vi "ShapeDectect.vi"(8 "error in (no error)":errorcluster, 9 "ROI Descriptor":T2, 10 "SetParameter":T4={"Enum_ShapeType"=enum."Circles", "MaxParticle"=1, "Descriptor"={"Set 1"=100.0, "Set 2"=10.0, "Set 3"=200.0, "Set 4"=10.0}, "Match Options"={"Rotation"=TRUE, "Scale"=FALSE, "Occlusion"=FALSE, "Range Settings"=[{"Match Constraints"=0, "Min"=0.0, "Max"=360.0}]}, "Curve Parameters"={"Extraction Mode"=0, "Edge Threshold"=75, "Edge Filter Size"=1, "Min Length"=25, "Row Search Step Size"=15, "Col Search Step Size"=15, "Max Endpoint Gap"=10, "Closed"=FALSE, "Subpixel"=FALSE}, " score"=500.0} {"score" format="%#_15g"; "Curve Parameters"."Extraction Mode" items=["Normal", "Uniform Regions"]; "Curve Parameters"."Edge Filter Size" items=["Fine", "Normal"]; "Match Options"."Range Settings"."Match Constraints" items=["Rotation Angle (degrees)", "Scale Factor (%)", "Occlusion (%)"]}, 11 "Image In":T3) -> (0 "error out":errorcluster, 1 "DectectItem":i32, 2 "ResultOut":variant, 3 "Image Out":T3)   [LabVIEW 2019]
uses:
  <vilib>/vision/Image Controls.llb/IMAQ Image.ctl
  Controls/ShapeDectect/Analysis_ShapeDectect_Parameter.ctl
  Controls/ShapeDectect/V_ShapeDectectFinalResult.ctl
  <vilib>/vision/NI_Vision_Development_Module.lvlib
panel:
  in  "Shapedectect Result Out":T1
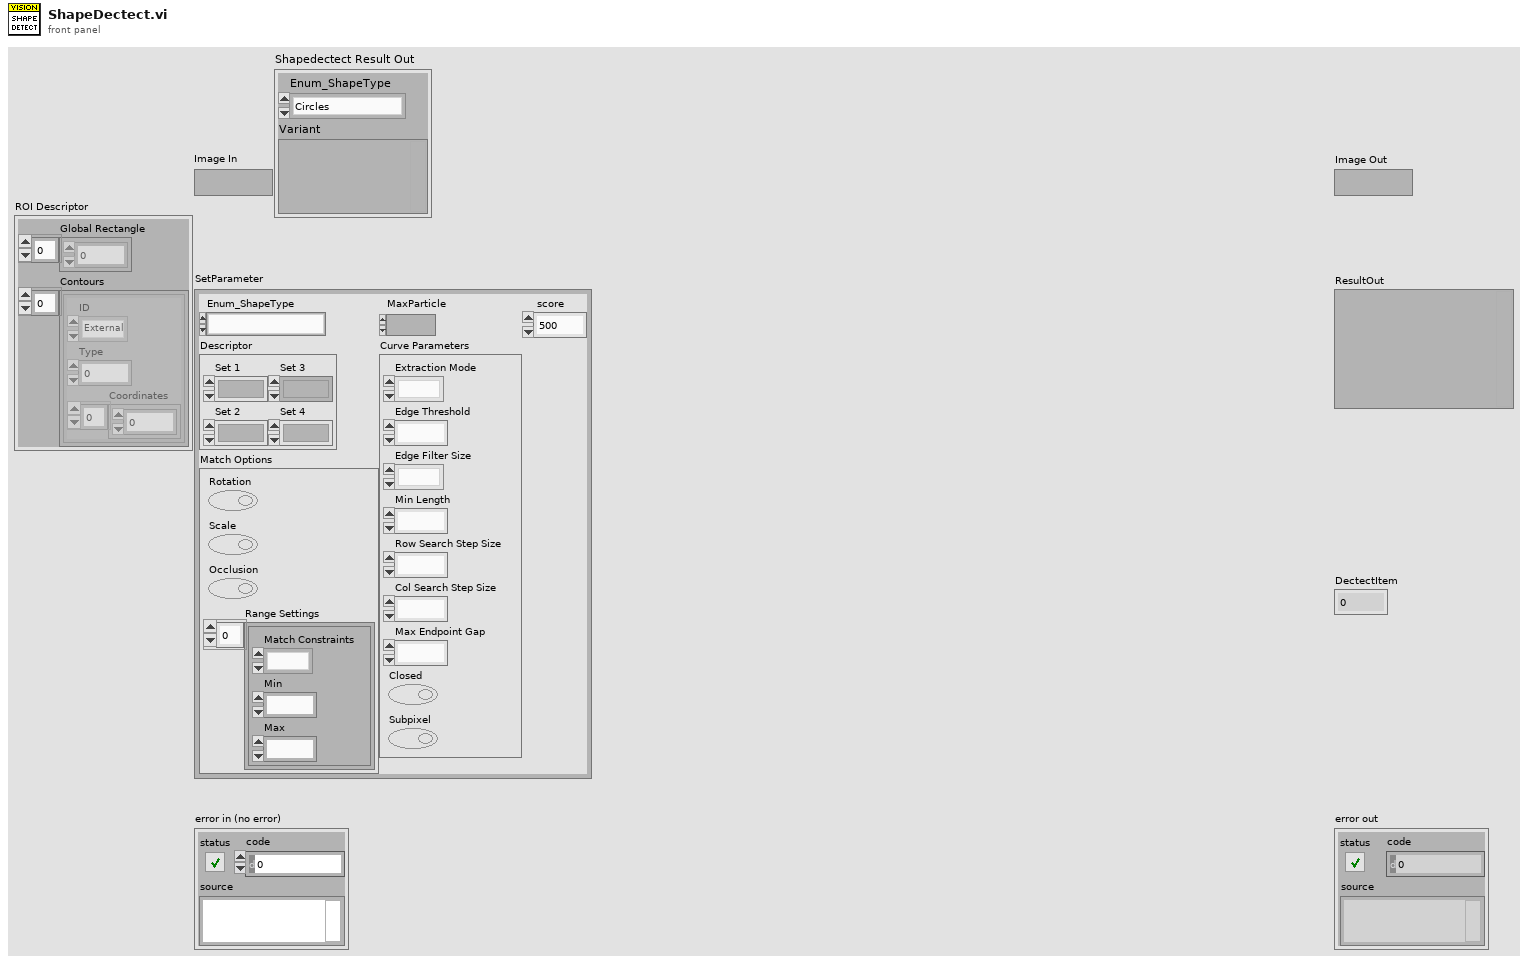
[diagram p1: front panel]
types:
  T1 = typedef "V_ShapeDectectFinalResult.ctl" = cluster{"Enum_ShapeType":enum16{"Circles", "Ellipses", "Lines", "Rectangles"}, "Variant":variant}
  T2 = cluster{"Global Rectangle":i32[], "Contours":cluster{"ID":enum32{"External", "Internal"}, "Type":u32, "Coordinates":i32[]}[]}
  T3 = typedef "IMAQ Image.ctl" = refnum<image>
  T4 = typedef "Analysis_ShapeDectect_Parameter.ctl" = cluster{"Enum_ShapeType":enum16{"Circles", "Ellipses", "Lines", "Rectangles"}, "MaxParticle":i32, "Descriptor":cluster{"Set 1":dbl, "Set 2":dbl, "Set 3":dbl, "Set 4":dbl}, "Match Options":cluster{"Rotation":bool, "Scale":bool, "Occlusion":bool, "Range Settings":cluster{"Match Constraints":u32, "Min":dbl, "Max":dbl}[]}, "Curve Parameters":cluster{"Extraction Mode":u32, "Edge Threshold":i32, "Edge Filter Size":u32, "Min Length":i32, "Row Search Step Size":i32, "Col Search Step Size":i32, "Max Endpoint Gap":i32, "Closed":bool, "Subpixel":bool}, " score":dbl}
  T5 = cluster{"Rectangles":cluster{"Corners":cluster{"X":sgl, "Y":sgl}[], "Angle":dbl, "Width":dbl, "Height":dbl, "Score":dbl}[], "Rectangles Calibrated":cluster{"Corners":cluster{"X":sgl, "Y":sgl}[], "Angle":dbl, "Width":dbl, "Height":dbl, "Score":dbl}[]}
  T6 = cluster{"Lines":cluster{"Start Point":cluster{"X":sgl, "Y":sgl}, "End Point":cluster{"X":sgl, "Y":sgl}, "Length":dbl, "Angle":dbl, "Score":dbl}[], "Lines Calibrated":cluster{"Start Point":cluster{"X":sgl, "Y":sgl}, "End Point":cluster{"X":sgl, "Y":sgl}, "Length":dbl, "Orientation":dbl, "Score":dbl}[]}
  T7 = cluster{"Pixel":cluster{"Position":cluster{"X":sgl, "Y":sgl}, "Angle":dbl, "Major Radius":dbl, "Minor Radius":dbl, "Score":dbl}[], "Ellipses (Calibrated)":cluster{"Position":cluster{"X":sgl, "Y":sgl}, "Orientation":dbl, "Major Radius":dbl, "Minor Radius":dbl, "Score":dbl}[]}
  T8 = cluster{"Circles":cluster{"Position":cluster{"X":sgl, "Y":sgl}, "Radius":dbl, "Score":dbl}[], "Circles (Calibrated)":cluster{"Position":cluster{"X":sgl, "Y":sgl}, "Radius":dbl, "Score":dbl}[]}
  T9 = enum16{"Circles", "Ellipses", "Lines", "Rectangles"}
  T10 = cluster{"Set 1":dbl, "Set 2":dbl, "Set 3":dbl, "Set 4":dbl}
  T11 = cluster{"Rotation":bool, "Scale":bool, "Occlusion":bool, "Range Settings":cluster{"Match Constraints":u32, "Min":dbl, "Max":dbl}[]}
  T12 = cluster{"Extraction Mode":u32, "Edge Threshold":i32, "Edge Filter Size":u32, "Min Length":i32, "Row Search Step Size":i32, "Col Search Step Size":i32, "Max Endpoint Gap":i32, "Closed":bool, "Subpixel":bool}
  T13 = cluster{"Position":cluster{"X":sgl, "Y":sgl}, "Radius":dbl, "Score":dbl}
  T14 = cluster{"Position":cluster{"X":sgl, "Y":sgl}, "Angle":dbl, "Major Radius":dbl, "Minor Radius":dbl, "Score":dbl}
  T15 = cluster{"Start Point":cluster{"X":sgl, "Y":sgl}, "End Point":cluster{"X":sgl, "Y":sgl}, "Length":dbl, "Angle":dbl, "Score":dbl}
  T16 = cluster{"Corners":cluster{"X":sgl, "Y":sgl}[], "Angle":dbl, "Width":dbl, "Height":dbl, "Score":dbl}
  T17 = cluster{"Position":cluster{"X":sgl, "Y":sgl}, "Radius":dbl, "Score":dbl}[]
  T18 = cluster{"Position":cluster{"X":sgl, "Y":sgl}, "Angle":dbl, "Major Radius":dbl, "Minor Radius":dbl, "Score":dbl}[]
  T19 = cluster{"Position":cluster{"X":sgl, "Y":sgl}, "Orientation":dbl, "Major Radius":dbl, "Minor Radius":dbl, "Score":dbl}[]
  T20 = cluster{"Start Point":cluster{"X":sgl, "Y":sgl}, "End Point":cluster{"X":sgl, "Y":sgl}, "Length":dbl, "Angle":dbl, "Score":dbl}[]
  T21 = cluster{"Start Point":cluster{"X":sgl, "Y":sgl}, "End Point":cluster{"X":sgl, "Y":sgl}, "Length":dbl, "Orientation":dbl, "Score":dbl}[]
  T22 = cluster{"Corners":cluster{"X":sgl, "Y":sgl}[], "Angle":dbl, "Width":dbl, "Height":dbl, "Score":dbl}[]
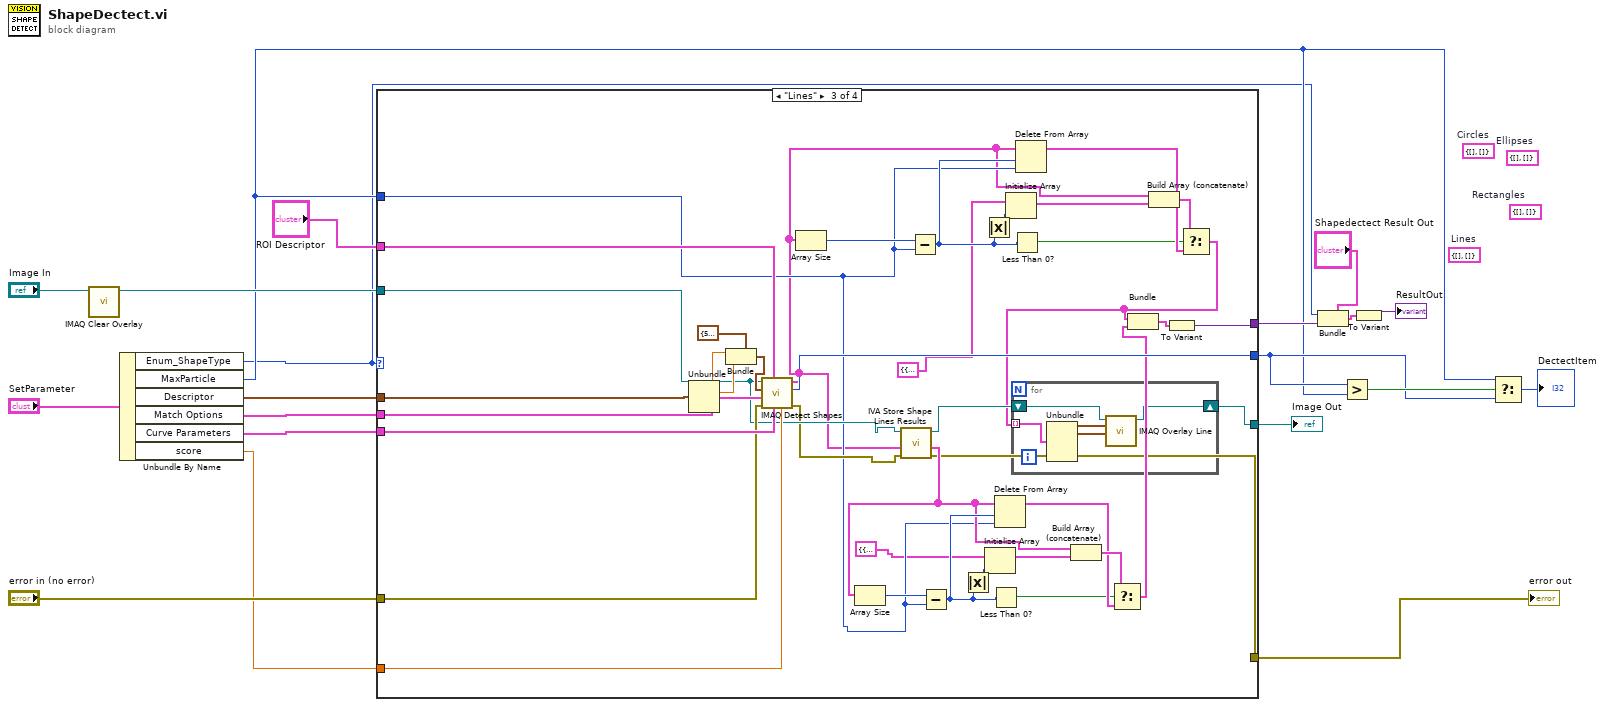
[diagram p0: block diagram]
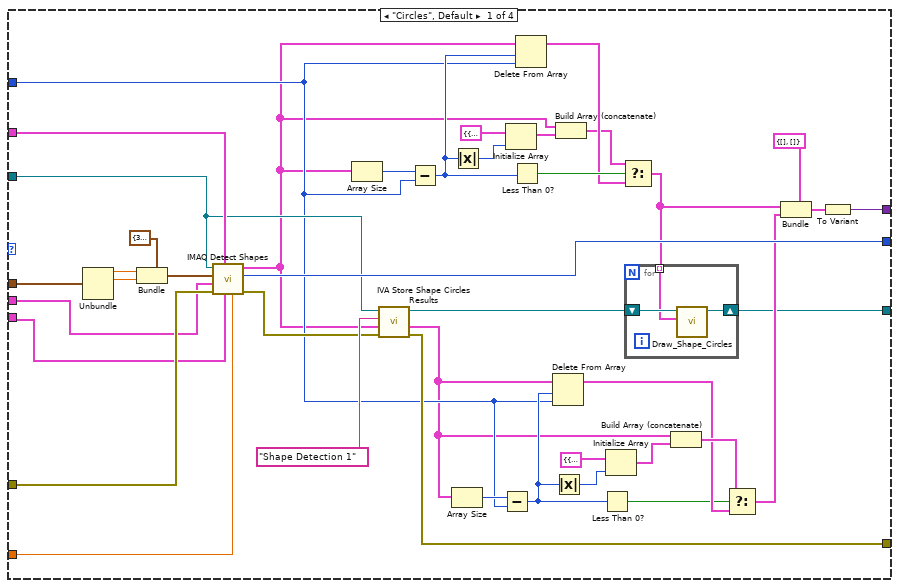
[diagram p2: hidden frame]
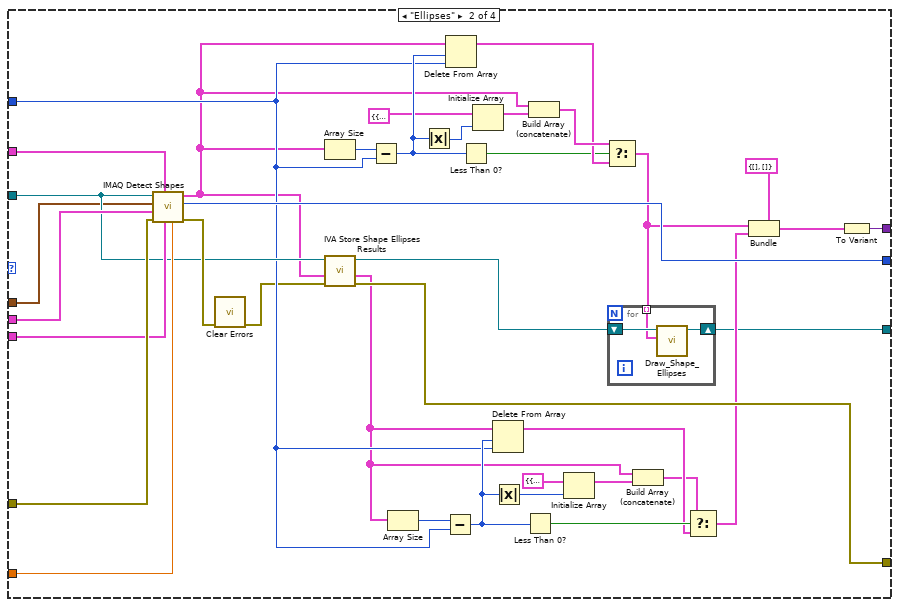
[diagram p3: hidden frame]
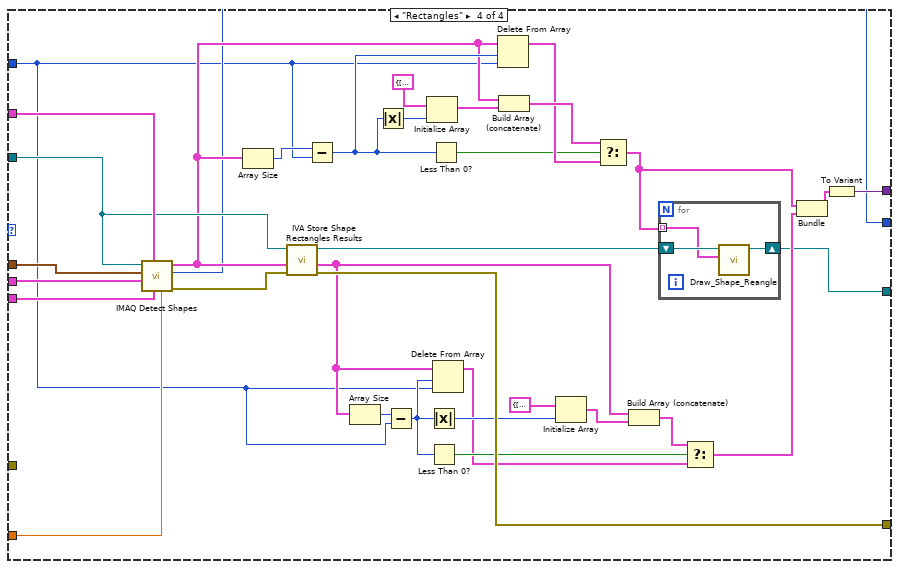
[diagram p4: hidden frame]
diagram:
  (unwired) T5 {"Rectangles"=[], "Rectangles Calibrated"=[]}  # Rectangles
  (unwired) T6 {"Lines"=[], "Lines Calibrated"=[]}  # Lines
  (unwired) T7 {"Pixel"=[], "Ellipses (Calibrated)"=[]}  # Ellipses
  (unwired) T8 {"Circles"=[], "Circles (Calibrated)"=[]}  # Circles
  n1 = call "IMAQ Clear Overlay"("Image"="Image In") -> ("Image Out"=w13:T3)  [unwired: 9 in, 1 out]
  n2 = Unbundle By Name("SetParameter") -> ("Enum_ShapeType"=w4:T9, "MaxParticle"=w9:i32, "Descriptor"=w8:T10, "Match Options"=w7:T11, "Curve Parameters"=w6:T12, "score"=w5:dbl)
  n3 = case shown="\"Lines\"" w4 {
    tunnel: "ROI Descriptor" -> [w59 w101 w143 w182]
    tunnel: w13 -> [w40 w85 w116 w168]
    tunnel: [w44 w100 w139 w151] -> w16
    tunnel: w7 -> [w22 w99 w142 w181]
    tunnel: "error in (no error)" -> [w61 w98 w124 _]
    tunnel: w6 -> [w21 w97 w141 w180]
    tunnel: w5 -> [w60 w96 w140 w179]
    tunnel: w8 -> [w57 w67 w138 w178]
    tunnel: [w53 w95 w133 w177] -> w19
    tunnel: [w41 w83 w109 w166] -> w11
    tunnel: w9 -> [w31 w74 w113 w150]
    tunnel: [w25 w70 w108 w154] -> w14
    frame "Circles", Default {
      n4 = Unbundle(w57) -> ("Set 1"=w56:dbl, "Set 2"=w55:dbl)  [unwired: 2 out]
      n5 = Bundle(cluster=cluster{"Min Radius":dbl, "Max Radius":dbl} {"Min Radius"=3.0, "Max Radius"=500.0} ("Circle Descriptor"), "Min Radius"=w56, "Max Radius"=w55) -> (w54:cluster{"Min Radius":dbl, "Max Radius":dbl})
      n6 = call-poly "IMAQ Detect Shapes"("Minimum match score"=w60, "Curve Parameters"=w21, "ROI Descriptor"=w59, "error in (no error)"=w61, "Match Options"=w22, "Circle Descriptor"=w54, "Image"=w40) -> ("error out"=w42:errorcluster, "Number of Matches Returned"=w44:i32, "Circles"=w24:T17)  [unwired: 2 out]
      n7 = Array Size(array=w24) -> (size(s)=w52:i32)
      n8 = call <vilib>:"IVA Store Shape Circles Results.vi"("error in (no error)"=w42, "Circles"=w24, "Step Name"="Shape Detection 1", "Image in"=w40) -> ("error out"=w41:errorcluster, "Circles (Calibrated)"=w30:T17, "Image dup"=w26:T3)  [unwired: 5 out]
      n9 = Subtract(x=w52, y=w31) -> (x-y=w49:i32)
      n10 = Array Size(array=w30) -> (size(s)=w32:i32)
      n11 = Absolute Value(x=w49) -> (abs(x)=w46:i32)
      n12 = Subtract(x=w32, y=w31) -> (x-y=w35:i32)
      n13 = Initialize Array(T13 {"Position"={"X"=0.0, "Y"=0.0}, "Radius"=0.0, "Score"=0.0} ("Circle Descriptor"), w46) -> (w48:T17)
      n14 = Less Than 0?(x=w49) -> (x < 0?=w51:bool)
      n15 = Delete From Array(array=w24, length=w49, index=w31) -> (array with subset deleted=w50:T17)  [unwired: 1 out]
      n16 = Delete From Array(array=w30, length=w35, index=w31) -> (array with subset deleted=w34:T17)  [unwired: 1 out]
      n17 = Absolute Value(x=w35) -> (abs(x)=w38:i32)
      n18 = Build Array (concatenate)(w24, w48) -> (w47:T17)
      n19 = Less Than 0?(x=w35) -> (x < 0?=w33:bool)
      n20 = Initialize Array(T13 {"Position"={"X"=0.0, "Y"=0.0}, "Radius"=0.0, "Score"=0.0} ("Circle Descriptor"), w38) -> (w36:T17)
      n21 = Select(t=w47, s=w51, f=w50) -> (s? t:f=w23:T17)
      n22 = for {
        shift-right: [w63] -> w25
        shift-left: w26 -> [w64]
        tunnel: w23 -> [w62] mode=indexing
        n23 = call "Draw_Shape_Circles.vi"("Circle Descriptor"=w62, "Image"=w64) -> ("Image Out"=w63:T3)  [unwired: 8 in, 1 out]
      }
      n24 = Build Array (concatenate)(w30, w36) -> (w37:T17)
      n25 = Select(t=w37, s=w33, f=w34) -> (s? t:f=w29:T17)
      n26 = Bundle(cluster=T8 {"Circles"=[], "Circles (Calibrated)"=[]}, "Circles"=w23, "Circles (Calibrated)"=w29) -> (w28:T8)
      n27 = To Variant(anything=w28) -> (Variant=w53:variant)
    }
    frame "Ellipses" {
      n28 = call-poly "IMAQ Detect Shapes"("Minimum match score"=w96, "Curve Parameters"=w97, "ROI Descriptor"=w101, "error in (no error)"=w98, "Match Options"=w99, "Ellipse Descriptor"=w67, "Image"=w85) -> ("error out"=w86:errorcluster, "Number of Matches Returned"=w100:i32, "Ellipses"=w69:T18)  [unwired: 2 out]
      n29 = call <vilib>:"Clear Errors.vi"("error in (no error)"=w86) -> ("error out"=w66:errorcluster)  [unwired: 5 in, 1 out]
      n30 = Array Size(array=w69) -> (size(s)=w88:i32)
      n31 = call <vilib>:"IVA Store Shape Ellipses Results.vi"("error in (no error)"=w66, "Ellipses"=w69, "Image in"=w85) -> ("error out"=w83:errorcluster, "Ellipses (Calibrated)"=w65:T19, "Image dup"=w84:T3)  [unwired: 1 in, 5 out]
      n32 = Subtract(x=w88, y=w74) -> (x-y=w91:i32)
      n33 = Array Size(array=w65) -> (size(s)=w81:i32)
      n34 = Absolute Value(x=w91) -> (abs(x)=w94:i32)
      n35 = Subtract(x=w81, y=w74) -> (x-y=w78:i32)
      n36 = Delete From Array(array=w69, length=w91, index=w74) -> (array with subset deleted=w90:T18)  [unwired: 1 out]
      n37 = Less Than 0?(x=w91) -> (x < 0?=w89:bool)
      n38 = Initialize Array(T14 {"Position"={"X"=0.0, "Y"=0.0}, "Angle"=0.0, "Major Radius"=0.0, "Minor Radius"=0.0, "Score"=0.0} ("Circle Descriptor"), w94) -> (w92:T18)
      n39 = Delete From Array(array=w65, length=w78, index=w74) -> (array with subset deleted=w79:T19)  [unwired: 1 out]
      n40 = Absolute Value(x=w78) -> (abs(x)=w75:i32)
      n41 = Less Than 0?(x=w78) -> (x < 0?=w80:bool)
      n42 = Build Array (concatenate)(w69, w92) -> (w93:T18)
      n43 = Initialize Array(T14 {"Position"={"X"=0.0, "Y"=0.0}, "Angle"=0.0, "Major Radius"=0.0, "Minor Radius"=0.0, "Score"=0.0} ("Circle Descriptor"), w75) -> (w77:T18)
      n44 = Select(t=w93, s=w89, f=w90) -> (s? t:f=w68:T18)
      n45 = for {
        shift-right: [w103] -> w70
        shift-left: w84 -> [w104]
        tunnel: w68 -> [w102] mode=indexing
        n46 = call "Draw_Shape_Ellipses.vi"("Ellipse Descriptor"=w102, "Image"=w104) -> ("Image Out"=w103:T3)  [unwired: 8 in, 1 out]
      }
      n47 = Build Array (concatenate)(w65, w77) -> (w76:T18)
      n48 = Select(t=w76, s=w80, f=w79) -> (s? t:f=w72:T19)
      n49 = Bundle(cluster=T7 {"Pixel"=[], "Ellipses (Calibrated)"=[]}, "Pixel"=w68, "Ellipses (Calibrated)"=w72) -> (w73:T7)
      n50 = To Variant(anything=w73) -> (Variant=w95:variant)
    }
    frame "Lines" {
      n51 = Unbundle(w138) -> ("Set 1"=w134:dbl, "Set 2"=w135:dbl)  [unwired: 2 out]
      n52 = Bundle(cluster=cluster{"Min Length":dbl, "Max Length":dbl} {"Min Length"=50.0, "Max Length"=500.0} ("Line Descriptor"), "Min Length"=w134, "Max Length"=w135) -> (w136:cluster{"Min Length":dbl, "Max Length":dbl})
      n53 = call-poly "IMAQ Detect Shapes"("Minimum match score"=w140, "Curve Parameters"=w141, "ROI Descriptor"=w143, "error in (no error)"=w124, "Match Options"=w142, "Line Descriptor"=w136, "Image"=w116) -> ("error out"=w115:errorcluster, "Number of Matches Returned"=w139:i32, "Lines"=w106:T20)  [unwired: 2 out]
      n54 = Array Size(array=w106) -> (size(s)=w126:i32)
      n55 = call <vilib>:"IVA Store Shape Lines Results.vi"("error in (no error)"=w115, "Lines"=w106, "Image in"=w116) -> ("error out"=w109:errorcluster, "Lines Calibrated"=w114:T21, "Image dup"=w107:T3)  [unwired: 1 in, 5 out]
      n56 = Array Size(array=w114) -> (size(s)=w117:i32)
      n57 = Subtract(x=w126, y=w113) -> (x-y=w129:i32)
      n58 = Subtract(x=w117, y=w113) -> (x-y=w120:i32)
      n59 = Absolute Value(x=w120) -> (abs(x)=w123:i32)
      n60 = Absolute Value(x=w129) -> (abs(x)=w132:i32)
      n61 = Initialize Array(T15 {"Start Point"={"X"=0.0, "Y"=0.0}, "End Point"={"X"=0.0, "Y"=0.0}, "Length"=0.0, "Angle"=0.0, "Score"=0.0} ("Circle Descriptor"), w123) -> (w121:T20)
      n62 = Less Than 0?(x=w120) -> (x < 0?=w118:bool)
      n63 = Delete From Array(array=w114, length=w120, index=w113) -> (array with subset deleted=w119:T21)  [unwired: 1 out]
      n64 = Initialize Array(T15 {"Start Point"={"X"=0.0, "Y"=0.0}, "End Point"={"X"=0.0, "Y"=0.0}, "Length"=0.0, "Angle"=0.0, "Score"=0.0} ("Circle Descriptor"), w132) -> (w130:T20)
      n65 = Less Than 0?(x=w129) -> (x < 0?=w127:bool)
      n66 = Delete From Array(array=w106, length=w129, index=w113) -> (array with subset deleted=w128:T20)  [unwired: 1 out]
      n67 = Build Array (concatenate)(w114, w121) -> (w122:T20)
      n68 = Select(t=w122, s=w118, f=w119) -> (s? t:f=w110:T21)
      n69 = Build Array (concatenate)(w106, w130) -> (w131:T20)
      n70 = Select(t=w131, s=w127, f=w128) -> (s? t:f=w105:T20)
      n71 = for {
        shift-right: [w148] -> w108
        shift-left: w107 -> [w147]
        tunnel: w105 -> [w146] mode=indexing
        n72 = Unbundle(w146) -> ("Start Point"=w145:cluster{"X":sgl, "Y":sgl}, "End Point"=w144:cluster{"X":sgl, "Y":sgl})  [unwired: 3 out]
        n73 = call "IMAQ Overlay Line"("End Point"=w144, "Start Point"=w145, "Image"=w147) -> ("Image Out"=w148:T3)  [unwired: 7 in, 1 out]
      }
      n74 = Bundle("Lines"=w105, "Lines Calibrated"=w110) -> (w111:T6)  [unwired: 1 in]
      n75 = To Variant(anything=w111) -> (Variant=w133:variant)
    }
    frame "Rectangles" {
      n76 = call-poly "IMAQ Detect Shapes"("Minimum match score"=w179, "Curve Parameters"=w180, "ROI Descriptor"=w182, "Match Options"=w181, "Rectangle Descriptor"=w178, "Image"=w168) -> ("error out"=w167:errorcluster, "Number of Matches Returned"=w151:i32, "Rectangles"=w153:T22)  [unwired: 1 in, 2 out]
      n77 = Array Size(array=w153) -> (size(s)=w170:i32)
      n78 = call <vilib>:"IVA Store Shape Rectangles Results.vi"("error in (no error)"=w167, "Rectangles"=w153, "Image in"=w168) -> ("error out"=w166:errorcluster, "Rectangles Calibrated"=w159:T22, "Image dup"=w155:T3)  [unwired: 1 in, 5 out]
      n79 = Subtract(x=w170, y=w150) -> (x-y=w173:i32)
      n80 = Array Size(array=w159) -> (size(s)=w160:i32)
      n81 = Absolute Value(x=w173) -> (abs(x)=w176:i32)
      n82 = Subtract(x=w160, y=w150) -> (x-y=w162:i32)
      n83 = Initialize Array(T16 {"Corners"=[], "Angle"=0.0, "Width"=0.0, "Height"=0.0, "Score"=0.0} ("Rectangle Descriptor"), w176) -> (w174:T22)
      n84 = Absolute Value(x=w162) -> (abs(x)=w165:i32)
      n85 = Less Than 0?(x=w162) -> (x < 0?=w161:bool)
      n86 = Less Than 0?(x=w173) -> (x < 0?=w171:bool)
      n87 = Delete From Array(array=w159, length=w162, index=w150) -> (array with subset deleted=w152:T22)  [unwired: 1 out]
      n88 = Delete From Array(array=w153, length=w173, index=w150) -> (array with subset deleted=w172:T22)  [unwired: 1 out]
      n89 = Build Array (concatenate)(w153, w174) -> (w175:T22)
      n90 = Initialize Array(T16 {"Corners"=[], "Angle"=0.0, "Width"=0.0, "Height"=0.0, "Score"=0.0} ("Rectangle Descriptor"), w165) -> (w163:T22)
      n91 = Select(t=w175, s=w171, f=w172) -> (s? t:f=w149:T22)
      n92 = Build Array (concatenate)(w159, w163) -> (w164:T22)
      n93 = for {
        shift-right: [w184] -> w154
        shift-left: w155 -> [w185]
        tunnel: w149 -> [w183] mode=indexing
        n94 = call "Draw_Shape_Reangle.vi"("Rectangle Descriptor"=w183, "Image"=w185) -> ("Image Out"=w184:T3)  [unwired: 8 in, 1 out]
      }
      n95 = Select(t=w164, s=w161, f=w152) -> (s? t:f=w158:T22)
      n96 = Bundle("Rectangles"=w149, "Rectangles Calibrated"=w158) -> (w156:T5)  [unwired: 1 in]
      n97 = To Variant(anything=w156) -> (Variant=w177:variant)
    }
  }
  "error out" <- w11
  "Image Out" <- w14
  n98 = Bundle(cluster="Shapedectect Result Out", "Enum_ShapeType"=w4, "Variant"=w19) -> (w2:T1)
  n99 = Greater?(x=w16, y=w9) -> (0:w17:bool)
  n100 = To Variant(anything=w2) -> (Variant=→"ResultOut":variant)
  n101 = Select(t=w9, s=w17, f=w16) -> (s? t:f=→"DectectItem":i32)
